vi "MSScript_SubVI_ListMSProcess.vi"() -> (0 "MSProcessList":string[](array[string]))   [LabVIEW 2018, in "MSScript.lvclass"]
uses:
  MSScript.lvclass
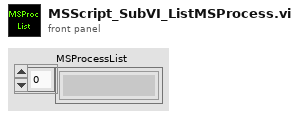
[diagram p1: front panel]
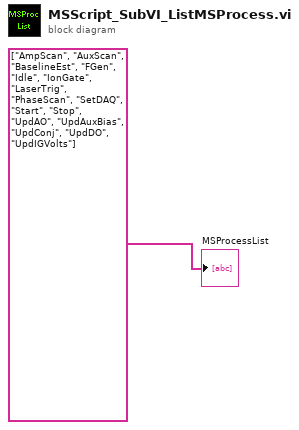
[diagram p0: block diagram]
diagram:
  "MSProcessList" <- string[] ["AmpScan", "AuxScan", "BaselineEst", "FGen", "Idle", "IonGate", "LaserTrig", "PhaseScan", "SetDAQ", "Start", "Stop", "UpdAO", "UpdAuxBias", "UpdConj", "UpdDO", "UpdIGVolts"]
